vi "Validate_Source.vi"(8 "error in (no error)":errorcluster, 10 "in build?":bool, 11 "Installer in":refnum<class "Installer.lvclass">) -> (0 "error out":errorcluster, 3 "Installer out":refnum<class "Installer.lvclass">)   [LabVIEW 2020, in "Installer.lvclass"]
uses:
  <vilib>/AppBuilder/IB_Classes/Installer/Installer.lvclass
  <vilib>/AppBuilder/IB_Classes/Installer/Installer.lvclass/Installer.ctl
  <vilib>/AppBuilder/IB_Classes/Source/IB_Source.lvclass
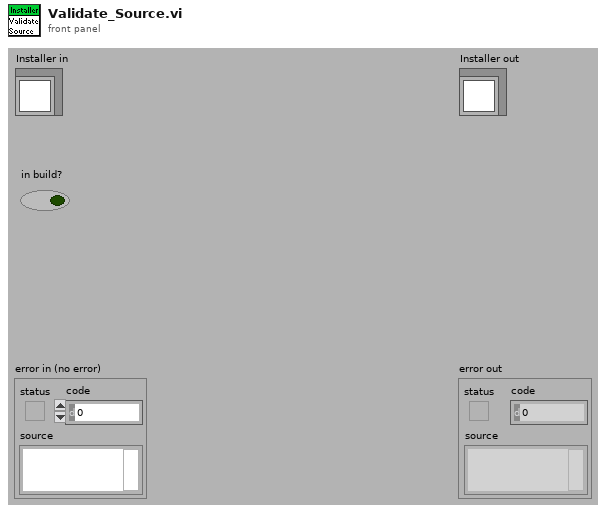
[diagram p1: front panel]
types:
  T1 = typedef "IB_Installer.ctl" = cluster{"Destination":refnum<class "IB_Destination.lvclass">[], "Source":refnum<class "IB_Source.lvclass">[], "buildObject":T2, "defaultDir":string, "platform":string, "author":string, "productName":string, "buildSpecName":string, "hide":bool, "requireLVDevSys":bool, "autoIncrement":bool, "includeError":bool, "readmeID":string, "buildLocation":path, "readmePath":path, "mediaSize":u16, "language":T3, "productVersion":T4, "preview":bool, "programmatic":bool, "progressBarEvents":T5, "userLog_Path":path, "shortcutAddresses":T7[], "EXE_Install Address":string, "EXE_Uninstall Address":string, "additional NIPaths":refnum<class "Dest_NI_NIPath.lvclass">[], "web service itemIDs":string[], "installerName":string}
  T2 = typedef "ItemRef.ctl" = u64
  T3 = typedef "CDK_sTypeDef_Languages.ctl" = u16
  T4 = typedef "CDK_sTypeDef_ProductVersion.ctl" = cluster{"Major":u8, "Minor":u8, "Update":u16}
  T5 = typedef "provcom_ProgressBar_Events.ctl" = cluster{"newJob":refnum<user-event>, "newItem":refnum<user-event>, "errorMsg":T6, "cancel":refnum<user-event>}
  T6 = typedef "mxLvBuildError.ctl" = refnum<user-event>
  T7 = typedef "CDK_sTypeDef_ShortcutAddress.ctl" = cluster{"file":string, "shortcut":string}
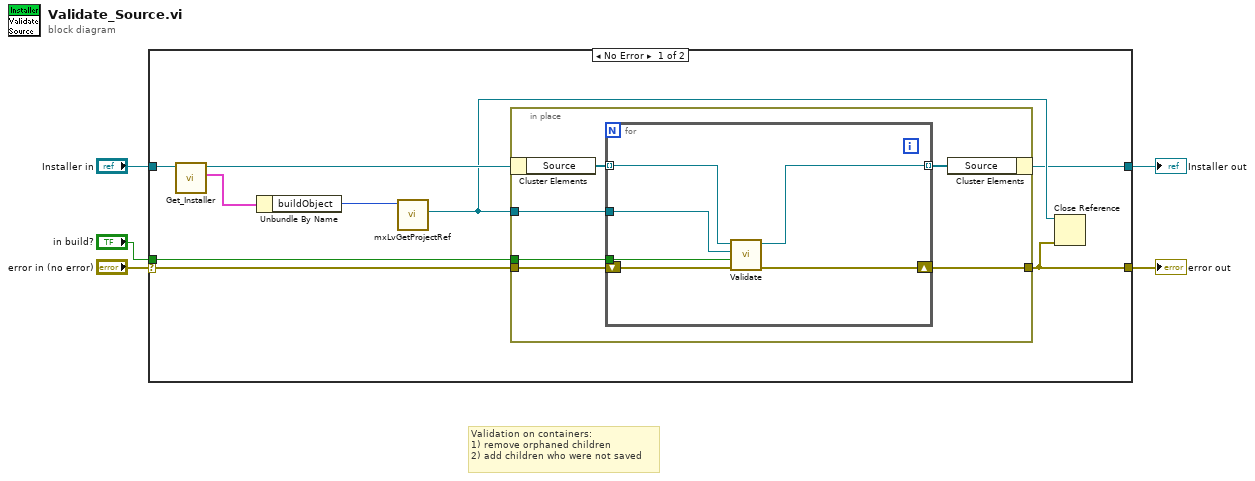
[diagram p0: block diagram]
diagram:
  # "Validation on containers:\n1) remove orphaned children\n2) add children who were not saved"
  n1 = case shown="No Error" "error in (no error)" {
    selector: "error in (no error)" -> [w11 w28]
    tunnel: [w6 w28] -> w4
    tunnel: [w7 w27] -> w2
    tunnel: "Installer in" -> [w13 w27]
    tunnel: "in build?" -> [w8 _]
    frame No Error {
      n2 = call <vilib>:"Get_Installer.vi"("Installer in"=w13) -> ("data"=w14:T1, "Installer out"=w12:refnum<class "Installer.lvclass">)  [unwired: 1 in, 8 out]
      n3 = Unbundle By Name(w14) -> ("buildObject"=w10:T2)
      n4 = call <resource>:"mxLvGetProjectRef.vi"("Item"=w10) -> ("Project Refnum"=w9:refnum<vi>)  [unwired: 1 in, 9 out]
      n5 = in-place {
        in-place-border: w9 -> [w18]
        in-place-border: [w17] -> w6
        in-place-border: w11 -> [w16]
        in-place-border: w8 -> [w15]
        n6 = in-place-cluster #1(w12) -> ("Source"=w20:refnum<class "IB_Source.lvclass">[])
        n7 = for {
          tunnel: w20 -> [w26] mode=indexing
          tunnel: [w25] -> w19 mode=indexing
          tunnel: w18 -> [w24]
          shift-right: [w23] -> w17
          shift-left: w16 -> [w22]
          tunnel: w15 -> [w21]
          n8 = call-dynamic "Validate.vi"("error in (no error)"=w22, "in build?"=w21, "proj refnum"=w24, "IB_Source in"=w26) -> ("error out"=w23:errorcluster, "IB_Source out"=w25:refnum<class "IB_Source.lvclass">)  [unwired: 6 out]
        }
        n9 = in-place-cluster #1("Source"=w19) -> (w7:refnum<class "Installer.lvclass">)
      }
      n10 = Close Reference(reference=w9, error in (no error)=w6) -> ()  [unwired: 1 out]
    }
    frame Error {
    }
  }
  "error out" <- w4
  "Installer out" <- w2
